vi "Wait until Axis is set.vi"(4 "Button Info":refnum<vi>, 6 "Axis Info":refnum<vi>, 8 "error in (no error)":errorcluster, 9 "Maximum?":bool, 10 "device ID in":refnum<k1>, 11 "Calibration Cluster in":T1) -> (0 "error out":errorcluster, 2 "Device ID out":refnum<k1>, 3 "Calibration Cluster out":T1, 5 "index":i32, 7 "Axis Array":i32[](array[numeric]))   [LabVIEW 2014]
uses:
  Controls/Controllers Clusters/Game Pad Calibration Cluster.ctl
  <vilib>/Utility/inputDevices.llb/joystickAcquire.vi
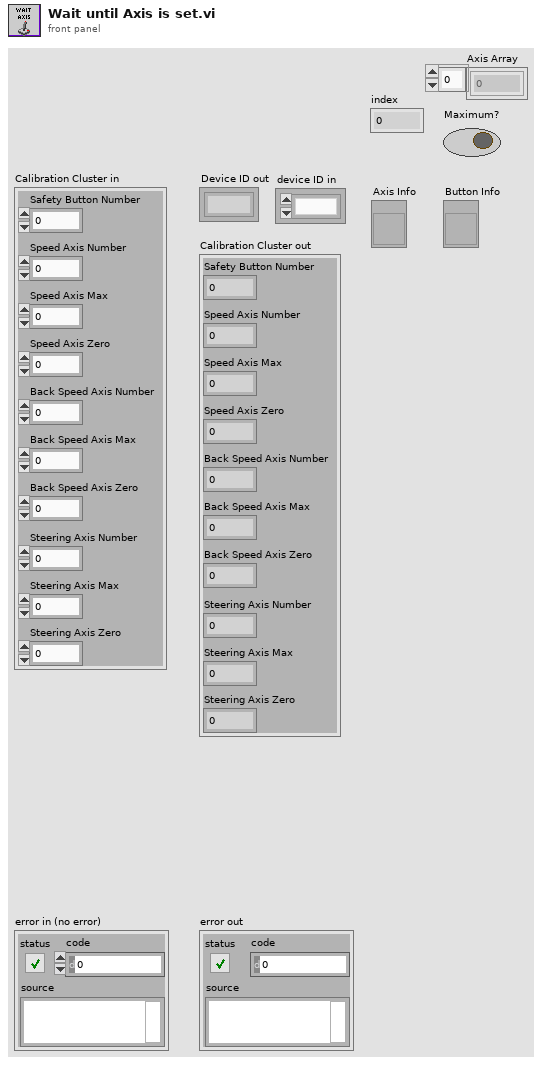
[diagram p1: front panel]
types:
  T1 = typedef "Game Pad Calibration Cluster.ctl" = cluster{"Safety Button Number":u8, "Speed Axis Number":u8, "Speed Axis Max":i32, "Speed Axis Zero":i32, "Back Speed Axis Number":u8, "Back Speed Axis Max":i32, "Back Speed Axis Zero":i32, "Steering Axis Number":u8, "Steering Axis Max":i32, "Steering Axis Zero":i32}
  T2 = cluster{"X axis":i32, "Y axis":i32, "Z axis":i32, "X axis rotation":i32, "Y axis rotation":i32, "Z axis rotation":i32, "U axis":i32, "V axis":i32}
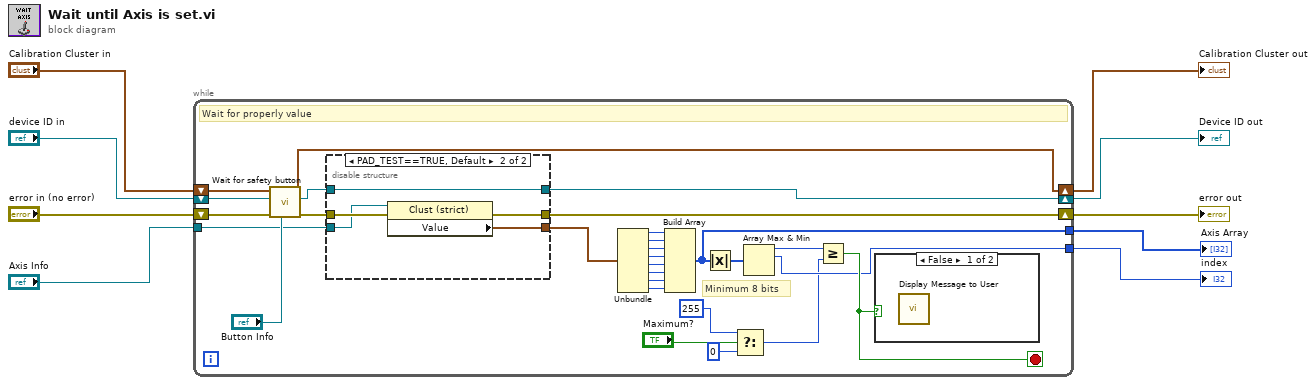
[diagram p0: block diagram]
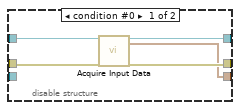
[diagram p2: hidden frame]
diagram:
  n1 = while {
    shift-right: [w17] -> w8
    shift-left: "device ID in" -> [w36]
    shift-right: [w18] -> w7
    shift-left: "Calibration Cluster in" -> [w34]
    shift-right: [w22] -> w9
    shift-left: "error in (no error)" -> [w37]
    tunnel: "Axis Info" -> [w20]
    tunnel: [w15] -> w2
    tunnel: [w14] -> w1
    stop <- w21 stop-if-true
    # "Minimum 8 bits"
    # "Wait for properly value"
    n2 = call "Wait for safety button.vi"("Button Info"="Button Info", "error in (no error)"=w37, "device ID in"=w36, "Calibration Cluster in"=w34) -> ("error out"=w33:errorcluster, "Refnum out"=w19:refnum<k1>, "Calibration Cluster out"=w18:T1)  [unwired: 5 in]
    n3 = disable-structure shown="PAD_TEST==TRUE, Default" {
      disable-tunnel: w33 -> [w42 w47]
      disable-tunnel: [w40 w46] -> w32
      disable-tunnel: [w41 w45] -> w22
      disable-tunnel: w20 -> [_ w44]
      disable-tunnel: w19 -> [w39 w43]
      disable-tunnel: [w38 w43] -> w17
      frame condition #0 {
        n4 = call-poly <vilib>:"Acquire Input Data.vi"("device ID"=w39, "error in (no error)"=w42) -> ("device ID"=w38:refnum<k1>, "axis info"=w40:T2, "error out"=w41:errorcluster)  [unwired: 13 in, 2 out]
      }
      frame condition #1 (active) {
        n5 = property on="Property Node" class="Clust (strict)"(reference=w44, error in=w47) -> (error out=w45:errorcluster, "Value"=w46:T2)  [unwired: 1 out]
      }
    }
    n6 = Unbundle(w32) -> ("X axis"=w31:i32, "Y axis"=w30:i32, "Z axis"=w29:i32, "X axis rotation"=w28:i32, "Y axis rotation"=w27:i32, "Z axis rotation"=w26:i32, "U axis"=w25:i32, "V axis"=w24:i32)
    n7 = Build Array(w31, w30, w29, w28, w27, w26, w25, w24) -> (w14:i32[])
    n8 = Absolute Value(x=w14) -> (abs(x)=w23:i32[])
    n9 = Select(t=255 ("y"), s="Maximum?", f=0) -> (s? t:f=w10:i32)
    n10 = Array Max & Min(array=w23) -> (max value=w16:i32, max index (indices)=w15:i32)  [unwired: 2 out]
    n11 = Greater Or Equal?(x=w16, y=w10) -> (x >= y?=w21:bool)
    n12 = case shown="False" w21 {
      frame False {
        n13 = call "Display Message to User"() -> ()  [unwired: 10 in, 2 out]
      }
      frame True {
      }
    }
  }
  "error out" <- w9
  "Device ID out" <- w8
  "Calibration Cluster out" <- w7
  "index" <- w2
  "Axis Array" <- w1
